vi "RT Main.vi"   [LabVIEW 2019]
uses:
  DataRecord.ctl
  trial type.ctl
  robot state.ctl
  commands.ctl
  <vilib>/Platform/TimedLoop/XDataNode/timing_clust.ctl
  <vilib>/Platform/TimedLoop/XDataNode/nitl_modes.ctl
  <vilib>/Platform/TimedLoop/XDataNode/wakeup.ctl
  RobotParams.ctl
  MvmtHistory.ctl
  TrialParams.ctl
  <vilib>/FPGAPlugInAG/cRIO-9053/niLvFpga_Open_cRIO-9053.vi
  <vilib>/rvi/interface/common/dynamic/niFpgaDynamicAddResources.vi
  <vilib>/Utility/error.llb/Error Cluster From Error Code.vi
  <vilib>/rvi/errors/niLvFpgaAdjustHostInterfaceError.vi
  <vilib>/Platform/TimedLoop/XDataNode/XDataNode.xnode
  <vilib>/rvi/interface/nirviOpenFPGA/nirviOpenFPGA.xnode
  FPGA Bitfiles/RobotNP_FPGATarget_FPGAmain_MtoEIOEvGZY.lvbitx
  FPGA main.vi
  <vilib>/rvi/interface/nirviReadWriteControl/nirviReadWriteControl.xnode
  <vilib>/Platform/TimedLoop/XDataNode/XDNodeRunTimeDep.lvlib
  <resource>/objmgr/ni.dex.rc
  <vilib>/rvi/interface/Simulation/niFpgaSimulationCallBeginRW.vi
  NiFpgaLv.dll
  <vilib>/ptbypt/NI_PtbyPt.lvlib
types:
  T1 = typedef "robot state.ctl" = enum16{"Hold", "Movement", "Homing", "Go somewhere", "Go home", "Disabled"}
  T2 = typedef "commands.ctl" = enum16{"TrialParams", "X home", "Y home", "Target X", "Target Y", "Enable drives", "Robot state", "Shut down", "Reward duration", "Start reward"}
  T3 = typedef "DataRecord.ctl" = cluster{"X":sgl, "Y":sgl, "MotorCurrent1":i16, "MotorCurrent2":i16, "TrialType":T4, "Angle":sgl, "FrameCnt1":i16, "FrameCnt2":i16, "Licking":bool, "Solenoid":bool, "robot state":T1}
  T4 = typedef "trial type.ctl" = enum8{"Linear", "2D aiming", "Two-part"}
  T5 = typedef "RobotParams.ctl" = cluster{"R1":dbl, "R2":dbl, "R3":dbl, "RadsPerCnt":dbl, "EncOffset1":i32, "EncOffset2":i32, "HomeX":dbl, "HomeY":dbl}
  T6 = typedef "XDNodeRunTimeDep.lvlib/timing_clust.ctl" = cluster{"Expected End [f-1]":u64, "Actual End [f-1]":u64, "Finished Late? [f-1]":bool, "Expected End [i-1]":u64, "Actual End [i-1]":u64, "Finished Late? [i-1]":bool, "Expected Start [i]":u64, "Actual Start [i]":u64, "Expected Start [f]":u64, "Actual Start [f]":u64, "Source Name":string, "Structure Name":string, "Period":i64, "Deadline":i64, "Offset":i64, "Start":i64, "Priority":i32, "Timeout":i32, "Mode":T7, "Wakeup Reason":T8, "Error":errorcluster, "Source Type":string, "Secondary Source Type":string, "Global End Time":u64, "Global Start Time":u64, "Frame Duration":u64, "Iteration Duration":u64, "Assigned CPU":i32, "I/O Scan Engine Mode":u32}
  T7 = typedef "XDNodeRunTimeDep.lvlib/nitl_modes.ctl" = enum32{"No Change", "Process missed periods, maintain original phase", "Discard missed periods, maintain original phase", "Process missed periods, ignore original phase", "Discard missed periods, ignore original phase"}
  T8 = typedef "XDNodeRunTimeDep.lvlib/wakeup.ctl" = enum32{"Normal", "Aborted", "Asynchronous wakeup", "Timing source error", "Timed loop error", "Timeout"}
  T9 = typedef "MvmtHistory.ctl" = cluster{"Xprev":dbl[], "Yprev":dbl[], "XerrSum":dbl, "XerrPrev":dbl, "OriginX":dbl, "OriginY":dbl, "FirstSegCur":bool, "FirstSegPrev":bool}
  T10 = typedef "TrialParams.ctl" = cluster{"Kp":dbl, "Bp":dbl, "Ip":dbl, "TrialType":T4, "Angle":dbl, "Viscosity":dbl, "Length":dbl, "MaxError":dbl, "TurnLength":dbl, "TurnAngle":dbl}
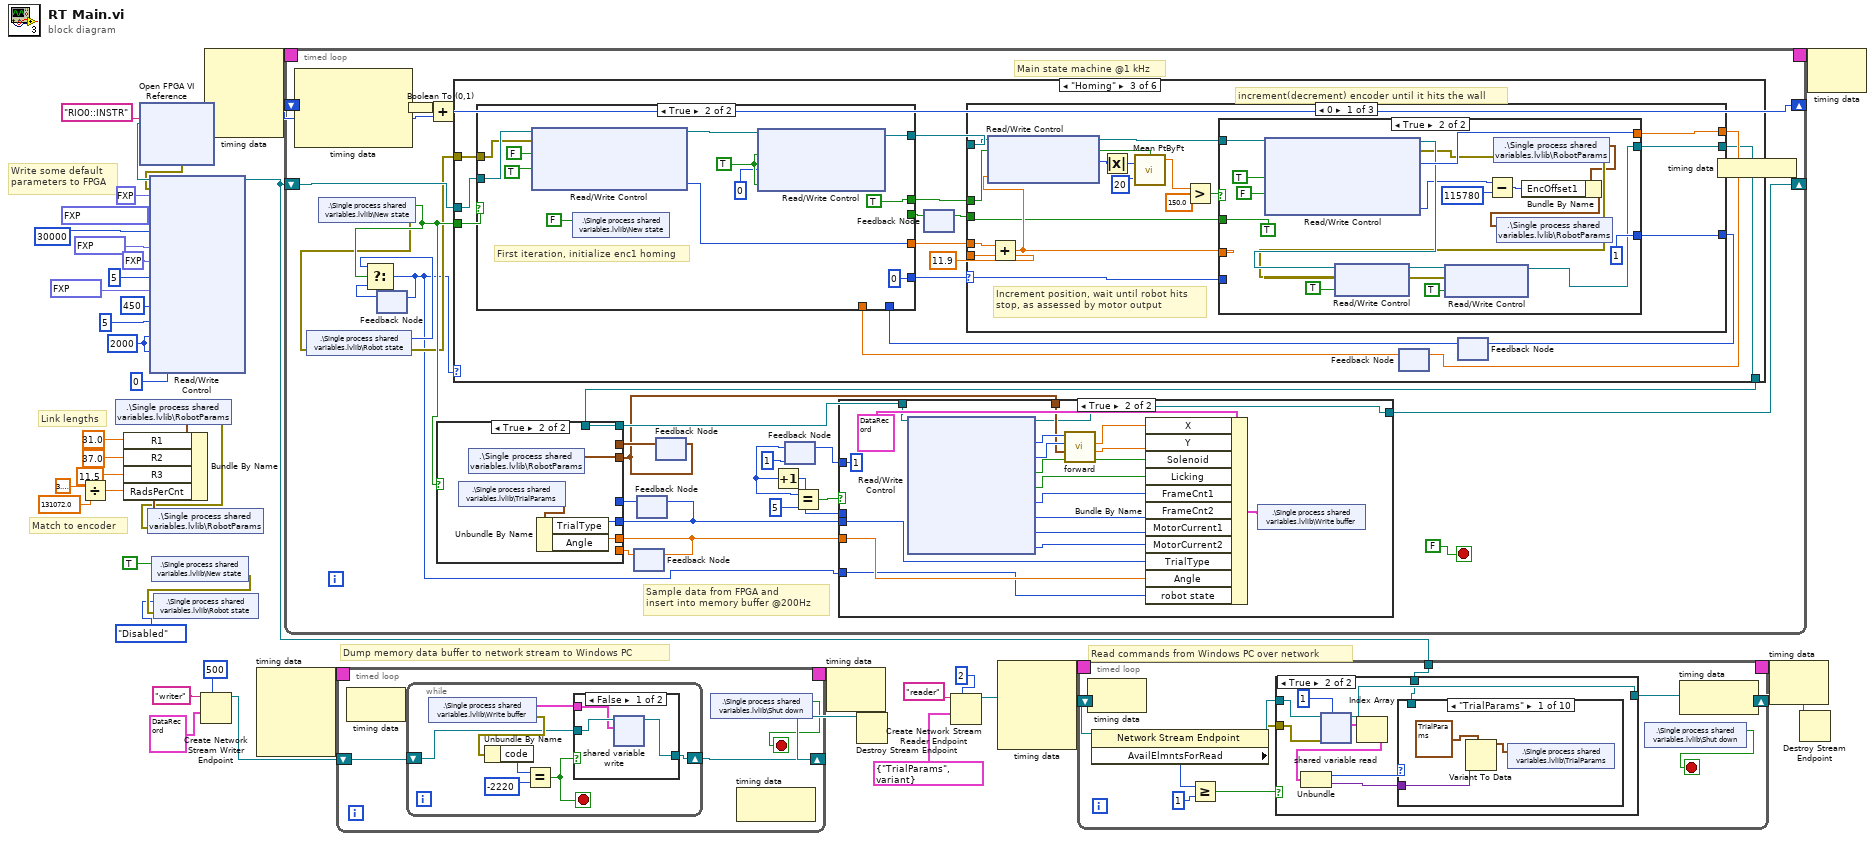
[diagram p0: block diagram]
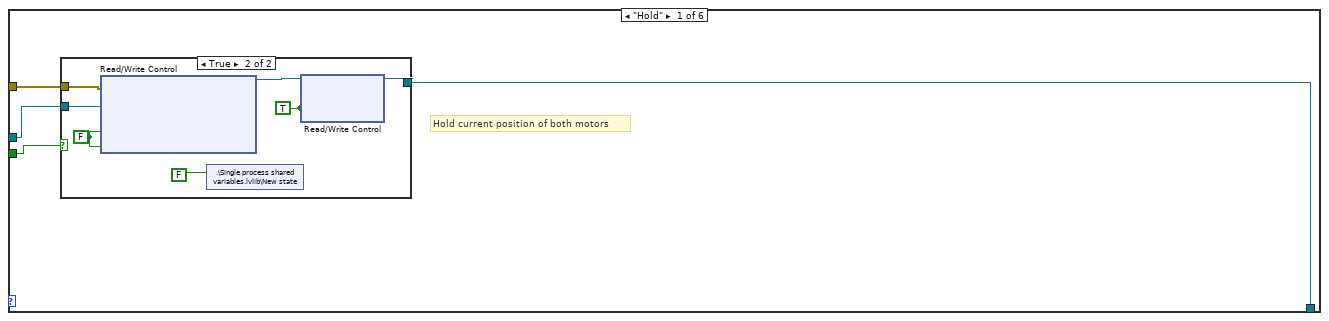
[diagram p5: hidden frame]
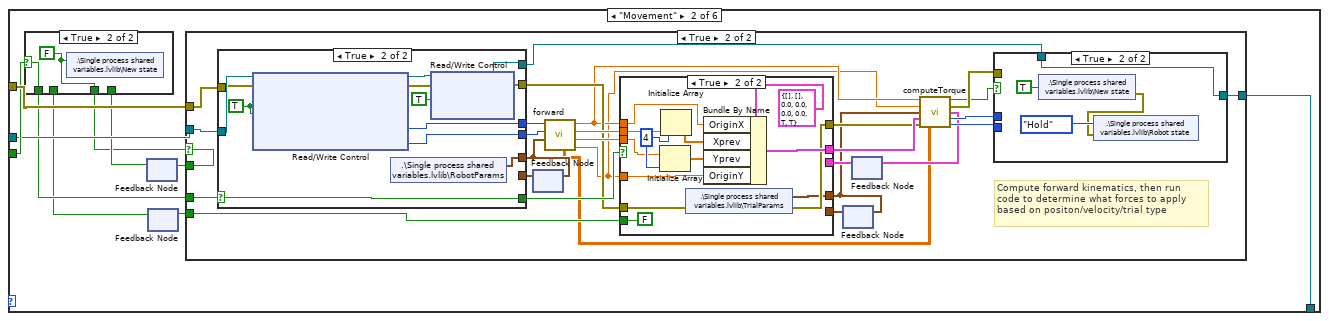
[diagram p7: hidden frame]
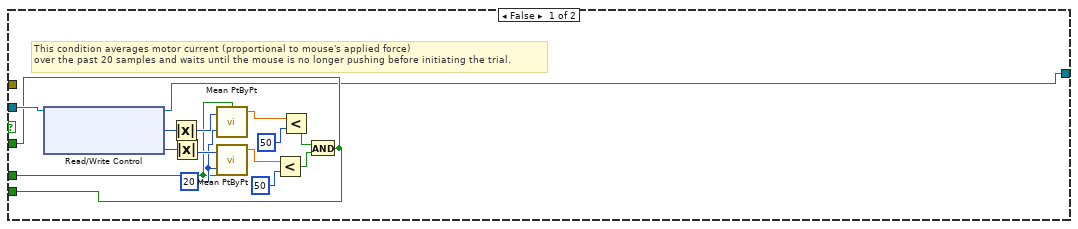
[diagram p8: hidden frame]
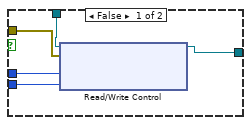
[diagram p10: hidden frame]
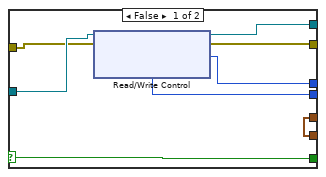
[diagram p11: hidden frame]
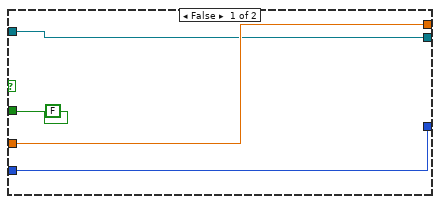
[diagram p13: hidden frame]
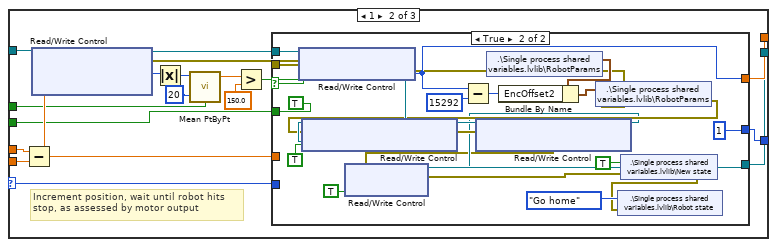
[diagram p14: hidden frame]
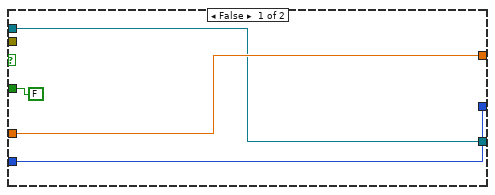
[diagram p15: hidden frame]
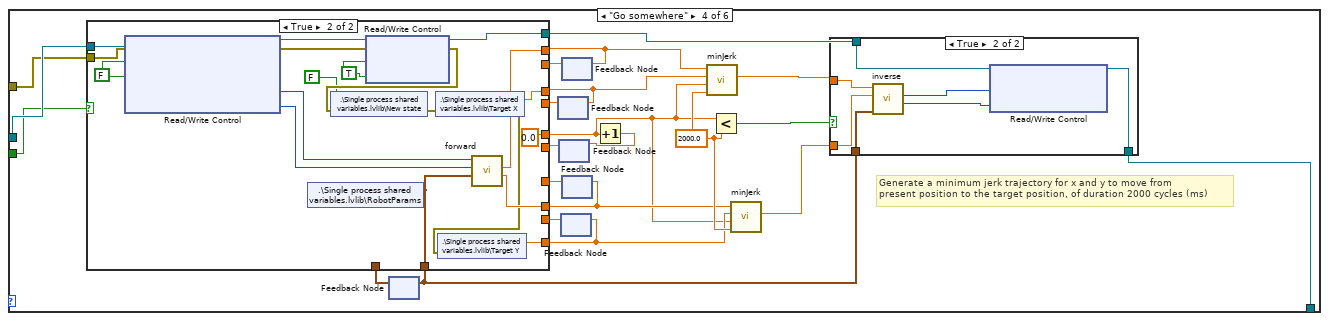
[diagram p18: hidden frame]
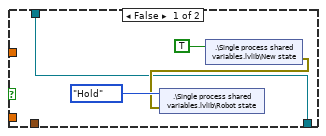
[diagram p19: hidden frame]
diagram:
  w29 = i16 2000 ("Current Min")
  # "Link lengths"
  # "Match to encoder"
  # "Write some default \nparameters to FPGA"
  # "Dump memory data buffer to network stream to Windows PC"
  # "Read commands from Windows PC over network"
  n1 = Divide(x=3.141592653589793, y=131072.0 ("Current Min")) -> (x/y=w8:dbl)
  n2 = shared-variable ".\\Single process shared variables.lvlib\\RobotParams"() -> (w5:T5, error out=w2:errorcluster)  [unwired: 1 in]
  n3 = Bundle By Name(cluster=w5, "R1"=31.0 ("Current Min"), "R2"=37.0 ("Current Min"), "R3"=11.5 ("Current Min"), "RadsPerCnt"=w8) -> (w12:T5)
  n4 = xnode "Open FPGA VI Reference"("resource name"="RIO0::INSTR") -> ("FPGA VI Reference Out"=w24:refnum<k20>, "error out"=w23:errorcluster)  [unwired: 1 in]
  n5 = shared-variable ".\\Single process shared variables.lvlib\\RobotParams"(w12, error in=w2) -> ()  [unwired: 1 out]
  n6 = xnode "Read/Write Control"("FPGA VI Reference In"=w24, "error in"=w23, "Pcurrent"=fxp<+/-,16,8> 4.0 ("Ki"), "Icurrent"=fxp<+/-,16,4> 0.050048828125 ("Ki"), "Imax"=i16 30000 ("Current Min"), "Kp"=fxp<+/-,16,10> 0.203125, "Kd"=fxp<+/-,16,10> 0.5, "Ipmax"=i16 5 ("Current Min"), "Ki"=fxp<+/-,16,10> 0.046875, "Current Limit"=i16 450 ("Current Min"), "Current Min"=i16 5, "pwm count 1"=w29, "pwm count 2"=w29, "Frame counter"=i16 0 ("Current Min")) -> ("FPGA VI Reference Out"=w36:refnum<k20>)  [unwired: 1 out]
  n7 = shared-variable ".\\Single process shared variables.lvlib\\New state"(TRUE) -> (error out=w38:errorcluster)  [unwired: 1 in]
  n8 = shared-variable ".\\Single process shared variables.lvlib\\Robot state"(robot_state."Disabled" ("Robot state"), error in=w38) -> ()  [unwired: 1 out]
  n9 = Create Network Stream Writer Endpoint(7:500, 9:T3 {"X"=0.0, "Y"=0.0, "MotorCurrent1"=0, "MotorCurrent2"=0, "TrialType"=enum."Linear", "Angle"=0.0, "FrameCnt1"=0, "FrameCnt2"=0, "Licking"=FALSE, "Solenoid"=FALSE, "robot state"=enum."Go somewhere"} ("DataRecord"), 11:"writer") -> (3:w15:refnum<k21>)  [unwired: 4 in, 1 out]
  n10 = node-c288() -> (w20:T6)  [unwired: 4 in]
  n11 = node-c288() -> (w18:T6)  [unwired: 4 in]
  n12 = timed-loop {
    timing: w20 -> [_]
    timing-out: [_] -> w19
    shift-right: [w51] -> _
    shift-left: w36 -> [w70]
    shift-right: [w58] -> _
    shift-left: _ -> [w57]
    stop <- FALSE stop-if-true
    # "Sample data from FPGA and \ninsert into memory buffer @200Hz"
    # "Main state machine @1 kHz"
    n13 = node-c288() -> (w60:bool)  [unwired: 1 in, 3 out]
    n14 = shared-variable ".\\Single process shared variables.lvlib\\New state"() -> (w63:bool, error out=w56:errorcluster)  [unwired: 1 in]
    n15 = shared-variable ".\\Single process shared variables.lvlib\\Robot state"(error in=w56) -> (w46:T1, error out=w55:errorcluster)
    n16 = feedback #1() -> (w44:T1)  [unwired: 1 in]
    n17 = Select(t=w46, s=w63, f=w44) -> (s? t:f=w45:T1)
    n18 = feedback-in #1(w45) -> ()
    n19 = Boolean To (0,1)(Boolean=w60) -> (0, 1=w59:i16)
    n20 = Add(x=w59, y=w57) -> (x+y=w58:i16)
    n21 = case shown="\"Homing\"" w45 {
      tunnel: w70 -> [w104 w118 w230 w358 w403 w408]
      tunnel: [w103 w122 w224 w353 w403 w407] -> w62
      tunnel: w63 -> [w102 w120 w220 w352 _ w406]
      tunnel: w55 -> [w101 w121 w219 w351 w399 w405]
      frame "Hold" {
        # "Hold current position of both motors"
        n22 = case shown="True" w102 {
          tunnel: w104 -> [w105 w112]
          tunnel: [w105 w107] -> w103
          tunnel: w101 -> [_ w111]
          frame False {
          }
          frame True {
            w108 = FALSE
            w110 = TRUE
            n23 = xnode "Read/Write Control"("FPGA VI Reference In"=w112, "error in"=w111, "Position / Current mode"=w108, "Position / Current mode 2"=w108) -> ("FPGA VI Reference Out"=w106:refnum<k20>)  [unwired: 3 out]
            n24 = shared-variable ".\\Single process shared variables.lvlib\\New state"(FALSE) -> ()  [unwired: 1 in, 1 out]
            n25 = xnode "Read/Write Control"("FPGA VI Reference In"=w106, "new mode"=w110, "new mode 2"=w110) -> ("FPGA VI Reference Out"=w107:refnum<k20>)  [unwired: 1 in, 1 out]
          }
        }
      }
      frame "Movement" {
        n26 = feedback #2() -> (w117:bool)  [unwired: 1 in]
        n27 = feedback #3() -> (w113:bool)  [unwired: 1 in]
        n28 = case shown="True" w120 {
          selector: w120 -> [_ w214]
          tunnel: w117 -> [w213 _]
          tunnel: [w213 w215] -> w115
          tunnel: [w212 w214] -> w114
          tunnel: w113 -> [w212 _]
          frame False {
          }
          frame True {
            w215 = FALSE
            n29 = shared-variable ".\\Single process shared variables.lvlib\\New state"(w215) -> ()  [unwired: 1 in, 1 out]
          }
        }
        n30 = case shown="True" w115 {
          selector: w115 -> [_ w161]
          tunnel: [w123 w158] -> w122
          tunnel: w121 -> [_ w146]
          tunnel: [w124 w161] -> w119
          tunnel: w118 -> [w134 w163]
          tunnel: [w124 w147] -> w116
          tunnel: w114 -> [w125 w162]
          frame False {
            w131 = i16 20
            # "This condition averages motor current (proportional to mouse's applied force)\nover the past 20 samples and waits until the mouse is no longer pushing before initiating the trial."
            n31 = xnode "Read/Write Control"("FPGA VI Reference In"=w134) -> ("FPGA VI Reference Out"=w123:refnum<k20>, "Current Feedback"=w137:i16, "Current Feedback 2"=w135:i16)  [unwired: 1 in, 1 out]
            n32 = Absolute Value(x=w137) -> (abs(x)=w133:i16)
            n33 = Absolute Value(x=w135) -> (abs(x)=w132:i16)
            n34 = call <vilib>:"Mean PtByPt.vi"("x"=w133, "sample length"=w131, "initialize"=w125) -> ("mean"=w129:dbl)  [unwired: 1 in, 1 out]
            n35 = call <vilib>:"Mean PtByPt.vi"("x"=w132, "sample length"=w131, "initialize"=w125) -> ("mean"=w128:dbl)  [unwired: 1 in, 1 out]
            n36 = Less?(x=w128, y=i16 50) -> (x < y?=w127:bool)
            n37 = Less?(x=w129, y=i16 50) -> (x < y?=w126:bool)
            n38 = And(x=w126, y=w127) -> (x .and. y?=w124:bool)
          }
          frame True {
            # "Compute forward kinematics, then run\ncode to determine what forces to apply \nbased on positon/velocity/trial type"
            n39 = feedback #4() -> (w154:T5)  [unwired: 1 in]
            n40 = case shown="True" w162 {
              selector: w162 -> [w193 w202]
              tunnel: w163 -> [w199 w208]
              tunnel: [w198 w209] -> w142
              tunnel: [w197 w205] -> w157
              tunnel: [w196 w204] -> w156
              tunnel: [w195 w203] -> w155
              tunnel: w154 -> [w195 _]
              tunnel: [w193 w202] -> w153
              tunnel: [w194 w201] -> w145
              tunnel: w146 -> [w192 w200]
              frame False {
                n41 = xnode "Read/Write Control"("FPGA VI Reference In"=w199, "error in"=w192) -> ("FPGA VI Reference Out"=w198:refnum<k20>, "error out"=w194:errorcluster, "Encoder Position"=w197:i32, "Encoder Position 2"=w196:i32)
              }
              frame True {
                w206 = TRUE
                w211 = TRUE
                n42 = xnode "Read/Write Control"("FPGA VI Reference In"=w208, "error in"=w200, "Position / Current mode"=w206, "Position / Current mode 2"=w206) -> ("FPGA VI Reference Out"=w210:refnum<k20>, "error out"=w207:errorcluster, "Encoder Position"=w205:i32, "Encoder Position 2"=w204:i32)
                n43 = shared-variable ".\\Single process shared variables.lvlib\\RobotParams"() -> (w203:T5)  [unwired: 1 in, 1 out]
                n44 = xnode "Read/Write Control"("FPGA VI Reference In"=w210, "error in"=w207, "new mode"=w211, "new mode 2"=w211) -> ("FPGA VI Reference Out"=w209:refnum<k20>, "error out"=w201:errorcluster)
              }
            }
            n45 = feedback-in #4(w155) -> ()
            n46 = call "forward.vi"("RobotParams"=w155, "Enc 2"=w156, "Enc 1"=w157) -> ("Y raw"=w139:dbl, "Y"=w152:dbl, "X"=w151:dbl, "X raw"=w140:dbl, "Jt"=w141:dbl[][])  [unwired: 4 in]
            n47 = feedback #5() -> (w143:T10)  [unwired: 1 in]
            n48 = feedback #6() -> (w148:T9)  [unwired: 1 in]
            n49 = case shown="True" w153 {
              selector: w153 -> [w168 _]
              tunnel: w139 -> [_ w180]
              tunnel: w140 -> [_ w179]
              tunnel: w152 -> [_ w178]
              tunnel: w151 -> [_ w177]
              tunnel: [w169 w174] -> w150
              tunnel: w148 -> [w169 _]
              tunnel: [w168 FALSE] -> w147
              tunnel: w145 -> [w166 w172]
              tunnel: [w166 w171] -> w144
              tunnel: [w167 w170] -> w138
              tunnel: w143 -> [w167 _]
              frame False {
              }
              frame True {
                w182 = 4
                n50 = Initialize Array(w178, w182) -> (w175:dbl[])
                n51 = Initialize Array(w177, w182) -> (w176:dbl[])
                n52 = shared-variable ".\\Single process shared variables.lvlib\\TrialParams"(error in=w172) -> (w170:T10, error out=w171:errorcluster)
                n53 = Bundle By Name(cluster=T9 {"Xprev"=[], "Yprev"=[], "XerrSum"=0.0, "XerrPrev"=0.0, "OriginX"=0.0, "OriginY"=0.0, "FirstSegCur"=TRUE, "FirstSegPrev"=TRUE} ("MvmtHistory"), "OriginX"=w179, "Xprev"=w176, "Yprev"=w175, "OriginY"=w180) -> (w174:T9)
              }
            }
            n54 = feedback-in #5(w138) -> ()
            n55 = call "computeTorque.vi"("X"=w140, "Y"=w139, "TrialParams"=w138, "MvmtHistory"=w150, "error in"=w144, "Jt"=w141) -> ("mvmtOver"=w159:bool, "error out"=w160:errorcluster, "MvmtHistoryOut"=w149:T9, "Torque 1"=w165:i16, "Torque 2"=w164:i16)  [unwired: 5 in]
            n56 = feedback-in #6(w149) -> ()
            n57 = case shown="True" w159 {
              tunnel: w165 -> [w187 _]
              tunnel: w164 -> [w186 _]
              tunnel: w160 -> [w185 _]
              tunnel: [w184 w188] -> w158
              tunnel: w142 -> [w183 w188]
              frame False {
                n58 = xnode "Read/Write Control"("FPGA VI Reference In"=w183, "error in"=w185, "Current Command"=w187, "Current Command 2"=w186) -> ("FPGA VI Reference Out"=w184:refnum<k20>)  [unwired: 1 out]
              }
              frame True {
                n59 = shared-variable ".\\Single process shared variables.lvlib\\New state"(TRUE) -> (error out=w189:errorcluster)  [unwired: 1 in]
                n60 = shared-variable ".\\Single process shared variables.lvlib\\Robot state"(robot_state."Hold" ("robot state"), error in=w189) -> ()  [unwired: 1 out]
              }
            }
          }
        }
        n61 = feedback-in #2(w119) -> ()
        n62 = feedback-in #3(w116) -> ()
      }
      frame "Homing" {
        # "increment(decrement) encoder until it hits the wall"
        n63 = feedback #7() -> (w216:bool)  [unwired: 1 in]
        n64 = feedback #8() -> (w225:dbl)  [unwired: 1 in]
        n65 = feedback #9() -> (w221:i32)  [unwired: 1 in]
        n66 = case shown="True" w220 {
          tunnel: w230 -> [w324 w336]
          tunnel: [w324 w334] -> w228
          tunnel: [w323 w333] -> w229
          tunnel: w225 -> [w323 _]
          tunnel: [w322 0] -> w223
          tunnel: w221 -> [w322 _]
          tunnel: w219 -> [_ w332]
          tunnel: [w321 TRUE] -> w218
          tunnel: w216 -> [w321 _]
          frame False {
          }
          frame True {
            w328 = TRUE
            # "First iteration, initialize enc1 homing"
            n67 = xnode "Read/Write Control"("FPGA VI Reference In"=w336, "error in"=w332, "Position / Current mode"=FALSE, "Position / Current mode 2"=TRUE) -> ("FPGA VI Reference Out"=w329:refnum<k20>, "Encoder Position"=w333:i32)  [unwired: 1 out]
            n68 = shared-variable ".\\Single process shared variables.lvlib\\New state"(FALSE) -> ()  [unwired: 1 in, 1 out]
            n69 = xnode "Read/Write Control"("FPGA VI Reference In"=w329, "new mode"=w328, "Current Command 2"=i16 0, "new mode 2"=w328) -> ("FPGA VI Reference Out"=w334:refnum<k20>)  [unwired: 1 in, 1 out]
          }
        }
        n70 = case shown="0" w223 {
          selector: w223 -> [w244 w276 w318]
          tunnel: w229 -> [w241 w286 _]
          tunnel: w228 -> [w247 w287 w320]
          tunnel: [w242 w284 w319] -> w226
          tunnel: 11.9 -> [w240 w285 w319]
          tunnel: [w238 w283 w320] -> w224
          tunnel: [w237 w281 w318] -> w222
          tunnel: w218 -> [w235 w274 w317]
          tunnel: [w234 w272 w317] -> w217
          frame 0 {
            # "Increment position, wait until robot hits\nstop, as assessed by motor output"
            n71 = Add(x=w241, y=w240) -> (x+y=w243:dbl)
            n72 = xnode "Read/Write Control"("FPGA VI Reference In"=w247, "Position Setpoint"=w243) -> ("FPGA VI Reference Out"=w239:refnum<k20>, "Current Feedback"=w246:i16)  [unwired: 1 in, 1 out]
            n73 = Absolute Value(x=w246) -> (abs(x)=w236:i16)
            n74 = call <vilib>:"Mean PtByPt.vi"("x"=w236, "sample length"=20, "initialize"=w235) -> ("mean"=w232:dbl)  [unwired: 1 in, 1 out]
            n75 = Greater?(x=w232, y=150.0) -> (0:w245:bool)
            n76 = case shown="True" w245 {
              tunnel: w244 -> [w251 _]
              tunnel: [w251 1] -> w237
              tunnel: w243 -> [w250 _]
              tunnel: [w250 w268] -> w242
              tunnel: w239 -> [w249 w269]
              tunnel: [w249 w252] -> w238
              tunnel: [FALSE TRUE] -> w234
              frame False {
              }
              frame True {
                n77 = xnode "Read/Write Control"("FPGA VI Reference In"=w269, "Position / Current mode"=TRUE, "Position / Current mode 2"=FALSE) -> ("FPGA VI Reference Out"=w265:refnum<k20>, "error out"=w262:errorcluster, "Encoder Position 2"=w268:i32, "Encoder Position"=w260:i32)  [unwired: 1 in]
                n78 = Subtract(x=w260, y=115780) -> (x-y=w256:i32)
                n79 = shared-variable ".\\Single process shared variables.lvlib\\RobotParams"(error in=w262) -> (w257:T5, error out=w261:errorcluster)
                n80 = xnode "Read/Write Control"("FPGA VI Reference In"=w265, "error in"=w261, "new mode"=TRUE) -> ("FPGA VI Reference Out"=w263:refnum<k20>, "error out"=w264:errorcluster)
                n81 = xnode "Read/Write Control"("FPGA VI Reference In"=w263, "error in"=w264, "new mode 2"=TRUE) -> ("FPGA VI Reference Out"=w252:refnum<k20>)  [unwired: 1 out]
                n82 = Bundle By Name(cluster=w257, "EncOffset1"=w256) -> (w258:T5)
                n83 = shared-variable ".\\Single process shared variables.lvlib\\RobotParams"(w258) -> ()  [unwired: 1 in, 1 out]
              }
            }
          }
          frame 1 {
            # "Increment position, wait until robot hits\nstop, as assessed by motor output"
            n84 = Subtract(x=w286, y=w285) -> (x-y=w288:dbl)
            n85 = xnode "Read/Write Control"("FPGA VI Reference In"=w287, "Position Setpoint 2"=w288) -> ("FPGA VI Reference Out"=w282:refnum<k20>, "error out"=w277:errorcluster, "Current Feedback 2"=w280:i16)  [unwired: 1 in]
            n86 = Absolute Value(x=w280) -> (abs(x)=w275:i16)
            n87 = call <vilib>:"Mean PtByPt.vi"("x"=w275, "sample length"=20, "initialize"=w274) -> ("mean"=w273:dbl)  [unwired: 1 in, 1 out]
            n88 = Greater?(x=w273, y=150.0) -> (0:w279:bool)
            n89 = case shown="True" w279 {
              tunnel: w276 -> [w292 _]
              tunnel: w288 -> [w291 _]
              tunnel: [w291 w306] -> w284
              tunnel: [w292 1] -> w281
              tunnel: [w290 w314] -> w283
              tunnel: w282 -> [w290 w313]
              tunnel: w277 -> [_ w310]
              tunnel: [FALSE TRUE] -> w272
              frame False {
              }
              frame True {
                n90 = xnode "Read/Write Control"("FPGA VI Reference In"=w313, "error in"=w310) -> ("FPGA VI Reference Out"=w309:refnum<k20>, "error out"=w304:errorcluster, "Encoder Position 2"=w306:i32)
                n91 = Subtract(x=w306, y=15292) -> (x-y=w303:i32)
                n92 = shared-variable ".\\Single process shared variables.lvlib\\RobotParams"(error in=w304) -> (w301:T5, error out=w297:errorcluster)
                n93 = Bundle By Name(cluster=w301, "EncOffset2"=w303) -> (w302:T5)
                n94 = shared-variable ".\\Single process shared variables.lvlib\\RobotParams"(w302, error in=w297) -> (error out=w300:errorcluster)
                n95 = xnode "Read/Write Control"("FPGA VI Reference In"=w309, "error in"=w300, "Position / Current mode 2"=TRUE) -> ("FPGA VI Reference Out"=w296:refnum<k20>, "error out"=w295:errorcluster)
                n96 = xnode "Read/Write Control"("FPGA VI Reference In"=w296, "error in"=w295) -> ("FPGA VI Reference Out"=w294:refnum<k20>, "error out"=w293:errorcluster)  [unwired: 1 out]
                n97 = xnode "Read/Write Control"("FPGA VI Reference In"=w294, "error in"=w293, "new mode 2"=TRUE) -> ("FPGA VI Reference Out"=w314:refnum<k20>, "error out"=w308:errorcluster)
                n98 = shared-variable ".\\Single process shared variables.lvlib\\New state"(TRUE, error in=w308) -> (error out=w299:errorcluster)
                n99 = shared-variable ".\\Single process shared variables.lvlib\\Robot state"(robot_state."Go home" ("robot state"), error in=w299) -> ()  [unwired: 1 out]
              }
            }
          }
          frame 2, Default {
          }
        }
        n100 = feedback-in #7(w217) -> ()
        n101 = feedback-in #8(w226) -> ()
        n102 = feedback-in #9(w222) -> ()
      }
      frame "Go somewhere" {
        w354 = 2000.0
        # "Generate a minimum jerk trajectory for x and y to move from\npresent position to the target position, of duration 2000 cycles (ms)"
        n103 = feedback #10() -> (w337:T5)  [unwired: 1 in]
        n104 = feedback #11() -> (w347:dbl)  [unwired: 1 in]
        n105 = feedback #12() -> (w345:dbl)  [unwired: 1 in]
        n106 = feedback #13() -> (w342:dbl)  [unwired: 1 in]
        n107 = feedback #14() -> (w349:dbl)  [unwired: 1 in]
        n108 = feedback #15() -> (w344:dbl)  [unwired: 1 in]
        n109 = case shown="True" w352 {
          tunnel: w358 -> [w376 w395]
          tunnel: [w376 w393] -> w338
          tunnel: [w373 w392] -> w343
          tunnel: [w371 w391] -> w348
          tunnel: [w375 0.0] -> w340
          tunnel: [w374 w389] -> w341
          tunnel: w345 -> [w375 _]
          tunnel: w342 -> [w374 _]
          tunnel: w344 -> [w373 _]
          tunnel: [w372 w388] -> w350
          tunnel: w351 -> [_ w384]
          tunnel: w349 -> [w372 _]
          tunnel: w347 -> [w371 _]
          tunnel: [w370 w377] -> w339
          tunnel: w337 -> [w370 _]
          frame False {
          }
          frame True {
            w382 = FALSE
            w394 = TRUE
            n110 = xnode "Read/Write Control"("FPGA VI Reference In"=w395, "error in"=w384, "Position / Current mode"=w382, "Position / Current mode 2"=w382) -> ("FPGA VI Reference Out"=w383:refnum<k20>, "error out"=w380:errorcluster, "Encoder Position"=w379:i32, "Encoder Position 2"=w378:i32)
            n111 = shared-variable ".\\Single process shared variables.lvlib\\RobotParams"() -> (w377:T5)  [unwired: 1 in, 1 out]
            n112 = xnode "Read/Write Control"("FPGA VI Reference In"=w383, "error in"=w380, "new mode"=w394, "new mode 2"=w394) -> ("FPGA VI Reference Out"=w393:refnum<k20>, "error out"=w387:errorcluster)
            n113 = shared-variable ".\\Single process shared variables.lvlib\\New state"(FALSE, error in=w387) -> (error out=w386:errorcluster)
            n114 = shared-variable ".\\Single process shared variables.lvlib\\Target X"(error in=w386) -> (w391:dbl, error out=w385:errorcluster)
            n115 = shared-variable ".\\Single process shared variables.lvlib\\Target Y"(error in=w385) -> (w389:dbl)  [unwired: 1 out]
            n116 = call "forward.vi"("RobotParams"=w377, "Enc 2"=w378, "Enc 1"=w379) -> ("Y"=w392:dbl, "X"=w388:dbl)  [unwired: 4 in, 3 out]
          }
        }
        n117 = feedback-in #10(w339) -> ()
        n118 = feedback-in #11(w348) -> ()
        n119 = feedback-in #13(w341) -> ()
        n120 = feedback-in #14(w350) -> ()
        n121 = feedback-in #15(w343) -> ()
        n122 = Increment(x=w340) -> (x+1=w346:dbl)
        n123 = feedback-in #12(w346) -> ()
        n124 = call "minJerk.vi"("tf"=w354, "t"=w340, "Xf"=w348, "Xi"=w350) -> ("Xnext"=w356:dbl)  [unwired: 7 in]
        n125 = Less?(x=w340, y=w354) -> (x < y?=w357:bool)
        n126 = call "minJerk.vi"("tf"=w354, "t"=w340, "Xf"=w341, "Xi"=w343) -> ("Xnext"=w355:dbl)  [unwired: 7 in]
        n127 = case shown="True" w357 {
          tunnel: w356 -> [_ w368]
          tunnel: w355 -> [_ w367]
          tunnel: [w359 w369] -> w353
          tunnel: w339 -> [_ w363]
          tunnel: w338 -> [w359 w364]
          frame False {
            n128 = shared-variable ".\\Single process shared variables.lvlib\\New state"(TRUE) -> (error out=w360:errorcluster)  [unwired: 1 in]
            n129 = shared-variable ".\\Single process shared variables.lvlib\\Robot state"(robot_state."Hold" ("robot state"), error in=w360) -> ()  [unwired: 1 out]
          }
          frame True {
            n130 = call "inverse.vi"("RobotParams"=w363, "Y"=w367, "X"=w368) -> ("Enc 2"=w365:i32, "Enc 1"=w366:i32)  [unwired: 7 in]
            n131 = xnode "Read/Write Control"("FPGA VI Reference In"=w364, "Position Setpoint"=w366, "Position Setpoint 2"=w365) -> ("FPGA VI Reference Out"=w369:refnum<k20>)  [unwired: 1 in, 1 out]
          }
        }
      }
      frame "Go home" {
        n132 = shared-variable ".\\Single process shared variables.lvlib\\Target X"(0.0, error in=w399) -> (error out=w398:errorcluster)
        n133 = shared-variable ".\\Single process shared variables.lvlib\\Target Y"(0.0, error in=w398) -> (error out=w401:errorcluster)
        n134 = shared-variable ".\\Single process shared variables.lvlib\\New state"(TRUE, error in=w401) -> (error out=w400:errorcluster)
        n135 = shared-variable ".\\Single process shared variables.lvlib\\Robot state"(robot_state."Go somewhere" ("robot state"), error in=w400) -> ()  [unwired: 1 out]
      }
      frame "Disabled", Default {
        # "Set motors to zero current output, then do nothing"
        n136 = case shown="True" w406 {
          tunnel: w408 -> [w409 w416]
          tunnel: [w409 w414] -> w407
          tunnel: w405 -> [_ w411]
          frame False {
          }
          frame True {
            w410 = TRUE
            w417 = i16 0
            w413 = TRUE
            n137 = xnode "Read/Write Control"("FPGA VI Reference In"=w416, "error in"=w411, "Current Command"=w417, "Position / Current mode"=w410, "Position / Current mode 2"=w410, "Current Command 2"=w417) -> ("FPGA VI Reference Out"=w415:refnum<k20>)  [unwired: 1 out]
            n138 = xnode "Read/Write Control"("FPGA VI Reference In"=w415, "new mode"=w413, "new mode 2"=w413) -> ("FPGA VI Reference Out"=w414:refnum<k20>, "error out"=w412:errorcluster)  [unwired: 1 in]
            n139 = shared-variable ".\\Single process shared variables.lvlib\\New state"(FALSE, error in=w412) -> ()  [unwired: 1 out]
          }
        }
      }
    }
    n140 = feedback #16() -> (w47:dbl)  [unwired: 1 in]
    n141 = feedback #17() -> (w49:T4)  [unwired: 1 in]
    n142 = feedback #18() -> (w54:T5)  [unwired: 1 in]
    n143 = case shown="True" w63 {
      tunnel: [w73 w78] -> w53
      tunnel: w54 -> [w73 _]
      tunnel: w62 -> [w74 w79]
      tunnel: [w74 w79] -> w61
      tunnel: [w72 w76] -> w50
      tunnel: [w71 w75] -> w48
      tunnel: w49 -> [w72 _]
      tunnel: w47 -> [w71 _]
      frame False {
      }
      frame True {
        n144 = shared-variable ".\\Single process shared variables.lvlib\\TrialParams"() -> (w77:T10)  [unwired: 1 in, 1 out]
        n145 = shared-variable ".\\Single process shared variables.lvlib\\RobotParams"() -> (w78:T5)  [unwired: 1 in, 1 out]
        n146 = Unbundle By Name(w77) -> ("TrialType"=w76:T4, "Angle"=w75:dbl)
      }
    }
    n147 = feedback-in #16(w48) -> ()
    n148 = feedback-in #17(w50) -> ()
    n149 = feedback-in #18(w53) -> ()
    n150 = feedback #19(1) -> (w66:i32)
    n151 = Increment(x=w66) -> (x+1=w65:i32)
    n152 = Equal?(x=w66, y=5) -> (x = y?=w68:bool)
    n153 = case shown="True" w68 {
      tunnel: w65 -> [w81 _]
      tunnel: [w81 1] -> w64
      tunnel: w53 -> [_ w96]
      tunnel: w61 -> [w80 w86]
      tunnel: [w80 w85] -> w51
      tunnel: w50 -> [_ w84]
      tunnel: w48 -> [_ w83]
      tunnel: w45 -> [_ w82]
      frame False {
      }
      frame True {
        n154 = xnode "Read/Write Control"("FPGA VI Reference In"=w86) -> ("FPGA VI Reference Out"=w85:refnum<k20>, "Encoder Position"=w98:i32, "Encoder Position 2"=w97:i32, "Solenoid open"=w95:bool, "Licking"=w94:bool, "Frame counter"=w93:i16, "Frame counter 2"=w92:i16, "Current Command"=w90:i16, "Current Command 2"=w91:i16)  [unwired: 1 in, 1 out]
        n155 = call "forward.vi"("RobotParams"=w96, "Enc 2"=w97, "Enc 1"=w98) -> ("Y"=w88:dbl, "X"=w89:dbl)  [unwired: 4 in, 3 out]
        n156 = Bundle By Name(cluster=T3 {"X"=0.0, "Y"=0.0, "MotorCurrent1"=0, "MotorCurrent2"=0, "TrialType"=enum."Linear", "Angle"=0.0, "FrameCnt1"=0, "FrameCnt2"=0, "Licking"=FALSE, "Solenoid"=FALSE, "robot state"=enum."Go somewhere"} ("DataRecord"), "X"=w89, "Y"=w88, "Solenoid"=w95, "Licking"=w94, "FrameCnt1"=w93, "FrameCnt2"=w92, "MotorCurrent1"=w90, "MotorCurrent2"=w91, "TrialType"=w84, "Angle"=w83, "robot state"=w82) -> (w87:T3)
        n157 = shared-variable ".\\Single process shared variables.lvlib\\Write buffer"(w87) -> ()  [unwired: 1 in, 1 out]
      }
    }
    n158 = feedback-in #19(w64) -> ()
    n159 = node-c288() -> ()  [unwired: 1 out]
  }
  n160 = timed-loop {
    shift-right: [w422] -> w13
    shift-left: w15 -> [w424]
    timing: w18 -> [_]
    timing-out: [_] -> w17
    stop <- w423 stop-if-true
    n161 = node-c288() -> ()  [unwired: 1 in, 1 out]
    n162 = while {
      shift-right: [w427] -> w422
      shift-left: w424 -> [w428]
      stop <- w426 stop-if-true
      n163 = shared-variable ".\\Single process shared variables.lvlib\\Write buffer"() -> (w430:T3, error out=w429:errorcluster)  [unwired: 1 in]
      n164 = Unbundle By Name(w429) -> ("code"=w425:i32)
      n165 = Equal?(x=w425, y=-2220) -> (x = y?=w426:bool)
      n166 = case shown="False" w426 {
        tunnel: w430 -> [w432 _]
        tunnel: w428 -> [w434 w435]
        tunnel: [w433 w435] -> w427
        frame False {
          n167 = shared-variable-write(w434, w432) -> (w433:refnum<k21>)  [unwired: 2 in, 2 out]
        }
        frame True {
        }
      }
    }
    n168 = shared-variable ".\\Single process shared variables.lvlib\\Shut down"() -> (w423:bool)  [unwired: 1 in, 1 out]
    n169 = node-c288() -> ()  [unwired: 1 in, 1 out]
  }
  n170 = node-c288(w17) -> ()  [unwired: 1 out]
  n171 = Destroy Stream Endpoint(11:w13) -> ()  [unwired: 1 in, 1 out]
  n172 = Create Network Stream Reader Endpoint(7:2, 9:cluster{T2, variant} {enum."TrialParams", variant}, 11:"reader") -> (3:w40:refnum<k21>)  [unwired: 4 in, 1 out]
  n173 = node-c288() -> (w43:T6)  [unwired: 4 in]
  n174 = timed-loop {
    shift-right: [w440] -> w39
    shift-left: w40 -> [w446]
    tunnel: w36 -> [w439]
    timing: w43 -> [_]
    timing-out: [_] -> w42
    stop <- w438 stop-if-true
    n175 = node-c288() -> ()  [unwired: 1 in, 1 out]
    n176 = property class="Network Stream Endpoint"(reference=w446) -> (reference out=w442:refnum<k21>, error out=w441:errorcluster, "AvailElmntsForRead"=w444:i32)  [unwired: 1 in]
    n177 = Greater Or Equal?(x=w444, y=1) -> (x >= y?=w443:bool)
    n178 = case shown="True" w443 {
      tunnel: w442 -> [w449 w458]
      tunnel: w441 -> [_ w457]
      tunnel: [w449 w455] -> w440
      tunnel: w439 -> [_ w454]
      frame False {
      }
      frame True {
        n179 = shared-variable-read(w458, w457, 1) -> (w455:refnum<k21>, w453:cluster{T2, variant}[])  [unwired: 1 in, 2 out]
        n180 = Index Array(array=w453) -> (element=w452:cluster{T2, variant})  [unwired: 1 in]
        n181 = Unbundle(w452) -> (w450:T2, w451:variant)
        n182 = case shown="\"TrialParams\"" w450 {
          tunnel: w451 -> [w461 w464 w467 w472 w475 w478 w486 _ w492 w496]
          tunnel: w454 -> [_ _ _ _ _ w481 _ _ w495 w499]
          frame "TrialParams" {
            n183 = Variant To Data(type=T10 {"Kp"=0.0, "Bp"=0.0, "Ip"=0.0, "TrialType"=enum."Linear", "Angle"=0.0, "Viscosity"=0.0, "Length"=0.0, "MaxError"=0.0, "TurnLength"=0.0, "TurnAngle"=0.0} ("TrialParams"), Variant=w461) -> (data=w459:T10)  [unwired: 1 in, 1 out]
            n184 = shared-variable ".\\Single process shared variables.lvlib\\TrialParams"(w459) -> ()  [unwired: 1 in, 1 out]
          }
          frame "X home" {
            n185 = Variant To Data(type=0.0, Variant=w464) -> (data=w462:dbl)  [unwired: 1 in, 1 out]
            n186 = shared-variable ".\\Single process shared variables.lvlib\\RobotParams"() -> (w465:T5)  [unwired: 1 in, 1 out]
            n187 = Bundle By Name(cluster=w465, "HomeX"=w462) -> (w466:T5)
            n188 = shared-variable ".\\Single process shared variables.lvlib\\RobotParams"(w466) -> ()  [unwired: 1 in, 1 out]
          }
          frame "Y home" {
            n189 = Variant To Data(type=0.0, Variant=w467) -> (data=w468:dbl)  [unwired: 1 in, 1 out]
            n190 = shared-variable ".\\Single process shared variables.lvlib\\RobotParams"() -> (w470:T5)  [unwired: 1 in, 1 out]
            n191 = Bundle By Name(cluster=w470, "HomeY"=w468) -> (w471:T5)
            n192 = shared-variable ".\\Single process shared variables.lvlib\\RobotParams"(w471) -> ()  [unwired: 1 in, 1 out]
          }
          frame "Target X" {
            n193 = Variant To Data(type=0.0, Variant=w472) -> (data=w473:dbl)  [unwired: 1 in, 1 out]
            n194 = shared-variable ".\\Single process shared variables.lvlib\\Target X"(w473) -> ()  [unwired: 1 in, 1 out]
          }
          frame "Target Y" {
            n195 = Variant To Data(type=0.0, Variant=w475) -> (data=w476:dbl)  [unwired: 1 in, 1 out]
            n196 = shared-variable ".\\Single process shared variables.lvlib\\Target Y"(w476) -> ()  [unwired: 1 in, 1 out]
          }
          frame "Enable drives" {
            n197 = Variant To Data(type=TRUE, Variant=w478) -> (data=w479:bool)  [unwired: 1 in, 1 out]
            n198 = case shown="False" w479 {
              tunnel: w481 -> [w483 w485]
              frame False {
                n199 = xnode "Read/Write Control"("FPGA VI Reference In"=w483, "Disable Drives"=TRUE) -> ()  [unwired: 1 in, 2 out]
              }
              frame True {
                n200 = xnode "Read/Write Control"("FPGA VI Reference In"=w485, "Enable Drives"=TRUE) -> ()  [unwired: 1 in, 2 out]
              }
            }
          }
          frame "Robot state" {
            n201 = Variant To Data(type=robot_state."Go somewhere" ("robot state"), Variant=w486) -> (data=w487:T1)  [unwired: 1 in, 1 out]
            n202 = shared-variable ".\\Single process shared variables.lvlib\\Robot state"(w487) -> (error out=w489:errorcluster)  [unwired: 1 in]
            n203 = shared-variable ".\\Single process shared variables.lvlib\\New state"(TRUE, error in=w489) -> ()  [unwired: 1 out]
          }
          frame "Shut down" {
            n204 = shared-variable ".\\Single process shared variables.lvlib\\Shut down"(TRUE) -> ()  [unwired: 1 in, 1 out]
          }
          frame "Reward duration" {
            n205 = Variant To Data(type=u32 0, Variant=w492) -> (data=w493:u32)  [unwired: 1 in, 1 out]
            n206 = xnode "Read/Write Control"("FPGA VI Reference In"=w495, "Reward"=w493) -> ()  [unwired: 1 in, 2 out]
          }
          frame "Start reward" {
            n207 = Variant To Data(type=TRUE, Variant=w496) -> (data=w497:bool)  [unwired: 1 in, 1 out]
            n208 = xnode "Read/Write Control"("FPGA VI Reference In"=w499, "Start reward"=w497) -> ()  [unwired: 1 in, 2 out]
          }
        }
      }
    }
    n209 = shared-variable ".\\Single process shared variables.lvlib\\Shut down"() -> (w438:bool)  [unwired: 1 in, 1 out]
    n210 = node-c288() -> ()  [unwired: 1 in, 1 out]
  }
  n211 = node-c288(w42) -> ()  [unwired: 1 out]
  n212 = Destroy Stream Endpoint(11:w39) -> ()  [unwired: 1 in, 1 out]
  n213 = node-c288(w19) -> ()  [unwired: 1 out]
